vi "Get Picture.vi"(8 "error in (no error)":errorcluster, 11 "Simple Case in":refnum<class "Simple Case.lvclass">) -> (0 "error out":errorcluster, 2 "Picture":picture, 3 "Simple Case out":refnum<class "Simple Case.lvclass">)   [LabVIEW 2020, in "Simple Case.lvclass"]
uses:
  Simple Case.lvclass
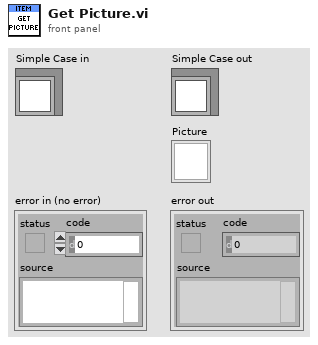
[diagram p1: front panel]
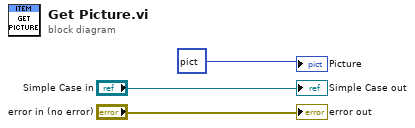
[diagram p0: block diagram]
diagram:
  "error out" <- "error in (no error)"
  "Simple Case out" <- "Simple Case in"
  "Picture" <- picture bytes[3230] ("new picture")
